vi "PotentiometerPacketParser.vi"(4 "Message":u8[](array[numeric])) -> (1 "Potentiometer Packet Out":T1)   [LabVIEW 2014]
uses:
  PotentiometerPacket.ctl
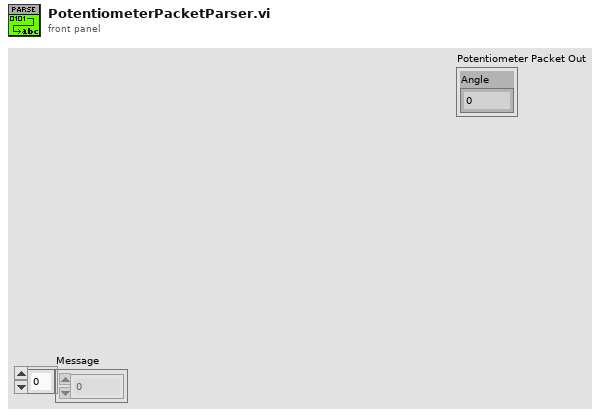
[diagram p1: front panel]
types:
  T1 = typedef "PotentiometerPacket.ctl" = cluster{"Angle":dbl}
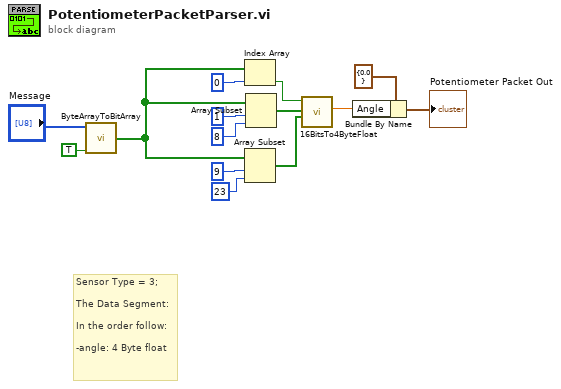
[diagram p0: block diagram]
diagram:
  # "Sensor Type = 3;\n\nThe Data Segment:\n\nIn the order follow:\n\n-angle: 4 Byte float"
  n1 = call "ByteArrayToBitArray.vi"("Flip Endian"=TRUE, "Byte Array In"="Message") -> ("Bit Array Out"=w1:bool[])  [unwired: 4 in]
  n2 = Index Array(array=w1, index=0) -> (element=w7:bool)
  n3 = Array Subset(array=w1, index=9, length=23) -> (w11:bool[])
  n4 = Array Subset(array=w1, index=1, length=8) -> (w14:bool[])
  n5 = call "16BitsTo4ByteFloat.vi"("Array"=w11, "Array 2"=w14, "Sign"=w7) -> ("Numeric"=w5:sgl)  [unwired: 6 in, 2 out]
  n6 = Bundle By Name(cluster=T1 {"Angle"=0.0} ("potentiometerPacket"), "Angle"=w5) -> (→"Potentiometer Packet Out":T1)
